vi "Read Teller Metadata.vi"(11 "Teller in":refnum<class "Teller.lvclass">) -> (2 "Teller Metadata":refnum<class "Teller Metadata.lvclass">)   [LabVIEW 2020, in "jettl.lvlib" / "Teller.lvclass"]
uses:
  Teller.lvclass
  Teller Metadata/Teller Metadata.lvclass
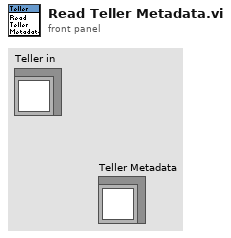
[diagram p1: front panel]
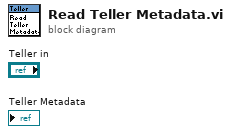
[diagram p0: block diagram]
diagram:
